vi "serial port list rev001.vi"() -> (4 "serial":u16(ring)=1 items=["COM1  (ASRL1  )", "COM3  (ASRL3  )", "COM15 (ASRL15  )", "", ""], 6 "I/O Array out":refnum<visa-resource-name>[](array[refnum])=["ASRL1::INSTR", "ASRL3::INSTR", "ASRL4::INSTR", ""], 8 "com port names":string[](array[string])=["ASRL1  (COM1 - Communications Port)", "ASRL3  (COM3)", "ASRL4  (COM4)", ""], 10 "com port count":i32)   [LabVIEW 2016]
panel:
  out "VISA resource name list out":refnum<visa-resource-name>="ASRL3::INSTR"
  out "return count":u32=4
  out "find list":string[](array[string])=["ASRL1::INSTR", "ASRL3::INSTR", "ASRL4::INSTR", "ASRL10::INSTR"]
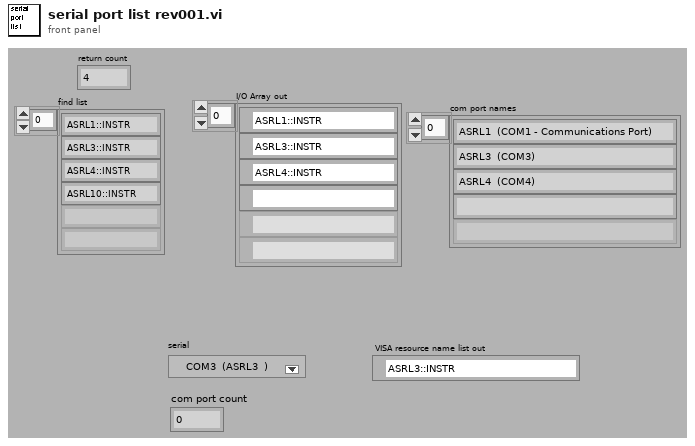
[diagram p1: front panel]
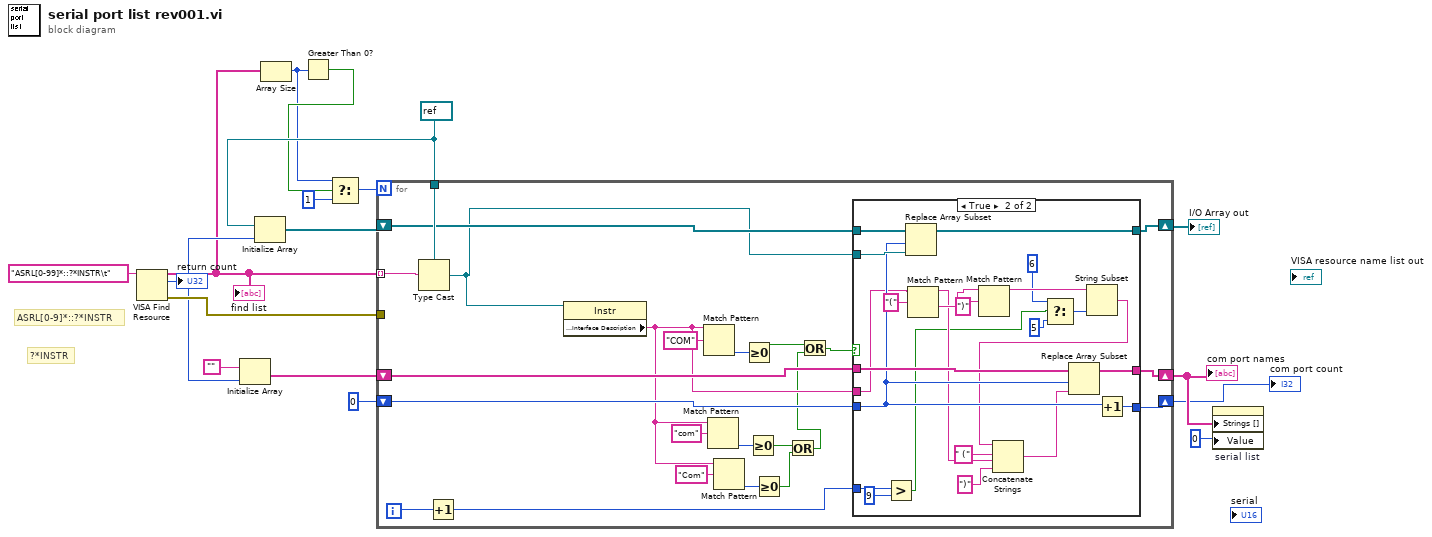
[diagram p0: block diagram]
diagram:
  w10 = refnum<visa-resource-name> refnum
  # "?*INSTR"
  # "ASRL[0-9]*::?*INSTR"
  n1 = VISA Find Resource(11:"ASRL[0-99]*::?*INSTR\t" ("expression (\"\")")) -> (0:w16:errorcluster, 2:w15:u32, 3:w5:string[])  [unwired: 1 in, 1 out]
  "find list" <- w5
  "return count" <- w15
  n2 = Initialize Array("", w15) -> (w12:string[])
  n3 = Initialize Array(w10, w15) -> (w13:refnum<visa-resource-name>[])
  n4 = Array Size(array=w5) -> (size(s)=w2:i32)
  n5 = Greater Than 0?(x=w2) -> (x > 0?=w3:bool)
  n6 = Select(t=w2, s=w3, f=1) -> (s? t:f=w4:i32)
  n7 = for {
    N: w4 -> [_]
    tunnel: w5 -> [w40] mode=indexing
    tunnel: w10 -> [w39]
    tunnel: w16 -> [_]
    shift-right: [w34] -> w7
    shift-left: w13 -> [w36]
    shift-right: [w32] -> w9
    shift-left: w12 -> [w33]
    shift-right: [w31] -> w6
    shift-left: 0 -> [w35]
    i -> [w20]
    n8 = Type Cast(type=w39, x=w40) -> (*(type *) &x=w18:refnum<visa-resource-name>)
    n9 = Increment(x=w20) -> (x+1=w19:i32)
    n10 = property class="Instr"(reference=w18) -> ("Interface Information:Interface Description"=w24:string)  [unwired: 1 in, 2 out]
    n11 = Match Pattern(string=w24, regular expression="COM") -> (offset past match=w37:i32)  [unwired: 4 out]
    n12 = Match Pattern(string=w24, regular expression="com") -> (offset past match=w25:i32)  [unwired: 4 out]
    n13 = Match Pattern(string=w24, regular expression="Com") -> (offset past match=w26:i32)  [unwired: 4 out]
    n14 = Greater Or Equal To 0?(x=w37) -> (x >= 0?=w28:bool)
    n15 = Greater Or Equal To 0?(x=w25) -> (x >= 0?=w21:bool)
    n16 = Greater Or Equal To 0?(x=w26) -> (x >= 0?=w23:bool)
    n17 = Or(x=w21, y=w23) -> (x .or. y?=w22:bool)
    n18 = Or(x=w28, y=w22) -> (x .or. y?=w29:bool)
    n19 = case shown="True" w29 {
      tunnel: w36 -> [w43 w66]
      tunnel: w35 -> [w41 w61]
      tunnel: w18 -> [_ w65]
      tunnel: [w43 w64] -> w34
      tunnel: w33 -> [w42 w63]
      tunnel: [w42 w62] -> w32
      tunnel: w24 -> [_ w54]
      tunnel: [w41 w60] -> w31
      tunnel: w19 -> [_ w49]
      frame False {
      }
      frame True {
        n20 = Greater?(x=w49, y=9) -> (0:w46:bool)
        n21 = Replace Array Subset(array=w66, new element=w65, index=w61) -> (w64:refnum<visa-resource-name>[])
        n22 = Match Pattern(string=w54, regular expression="(") -> (before substring=w51:string, after substring=w58:string)  [unwired: 3 out]
        n23 = Match Pattern(string=w58, regular expression=")") -> (before substring=w52:string)  [unwired: 4 out]
        n24 = Select(t=6 ("length (rest)"), s=w46, f=5) -> (s? t:f=w47:i32)
        n25 = String Subset(string=w52, length (rest)=w47) -> (substring=w50:string)  [unwired: 1 out]
        n26 = Concatenate Strings(w50, " (" ("regular expression"), w51, ")") -> (w53:string)
        n27 = Replace Array Subset(array=w63, new element=w53, index=w61) -> (w62:string[])
        n28 = Increment(x=w61) -> (x+1=w60:i32)
      }
    }
  }
  "I/O Array out" <- w7
  "com port names" <- w9
  "com port count" <- w6
  n29 = property on="serial list" class="Ring (strict)"("Strings []"=w9, "Value"=0) -> ()  [unwired: 2 in, 2 out]
